vi "IO_TEST_TankControl18V7.vi"() -> ()   [LabVIEW 2024]
uses:
  Control Definitions/Def_Status18v7.ctl
  <vilib>/Instr/_visa.llb/VISA Configure Serial Port (Instr).vi
  LabVIEW_InstrDriver_forLK-G3000_ver1_0_1_0/32bit/Keyence LK-G3000/Keyence LK-G3000.lvlib
panel:
  out "Elapsed":dbl format="%#.2g"
  out "Rate In/sec":dbl=nan format="%#.4g"
  in  "Reset":bool
  in  "Start":bool
  in  "Time (sec)":dbl=30.0
  in  "Laser ON":bool=TRUE
  out "Level PV":dbl(slide)=7.1220598220825195 scale=0.0..10.0
  out "Laser Raw":sgl=2.4953
  in  "Inputs":T1={"Fill!Drain"=TRUE, "Speed"=2, "Send Msg"=FALSE, "Write Buf"="GO"} {"Speed" scale=0.0..100.0}
  out "Outputs":T3={"Status"=[TRUE, FALSE, FALSE, FALSE, FALSE, FALSE, FALSE, FALSE, FALSE, FALSE, FALSE, FALSE, FALSE, FALSE, FALSE, FALSE, FALSE, FALSE, FALSE, FALSE, FALSE, FALSE, FALSE, FALSE, FALSE, FALSE, FALSE, FALSE, FALSE, FALSE, FALSE, FALSE], "Match"=-1, "Rx Speed"=".+64", "Tx"=FALSE}
  in  "Sens Reply":bool
  out "TX Buf":string="D0\r"
  in  "Send Reply":string
  out "read buffer ASC":string="!1\r\n"
  in  "Exit":bool
  # "Use this Timer section\nto measure the Level dl/dt"
  # "Laser ON When Laser\nis on Line."
  # "Use if off line to generate\na test Reply to Write msg"
  # "Fill"
  # "Drain"
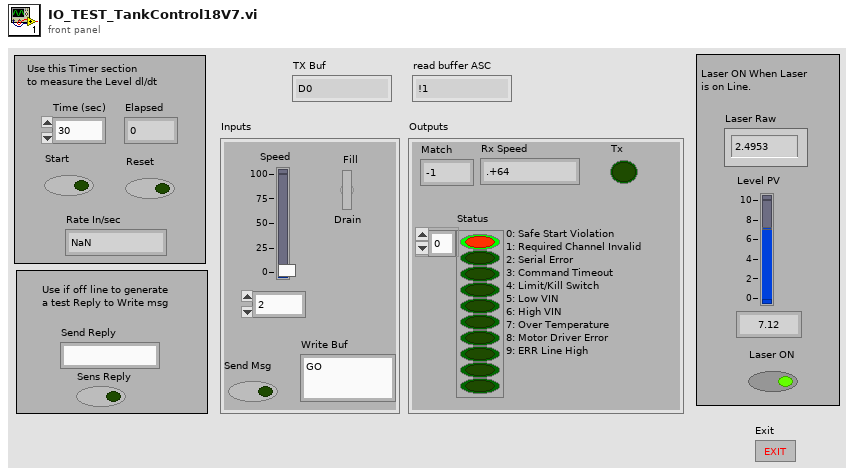
[diagram p1: front panel]
types:
  T1 = cluster{"Fill!Drain":bool, "Speed":i16, "Send Msg":bool, "Write Buf":string}
  T2 = typedef "Def_Status18v7.ctl" = bool[]
  T3 = cluster{"Status":T2, "Match":i32, "Rx Speed":string, "Tx":bool}
  T4 = typedef "Keyence LK-G3000.lvlib/LKIF_FLOATVALUE.ctl" = cluster{"LKIF_FLOATRESULT":T5, "Value":sgl}
  T5 = typedef "Keyence LK-G3000.lvlib/LKIF_FLOATRESULT.ctl" = i32
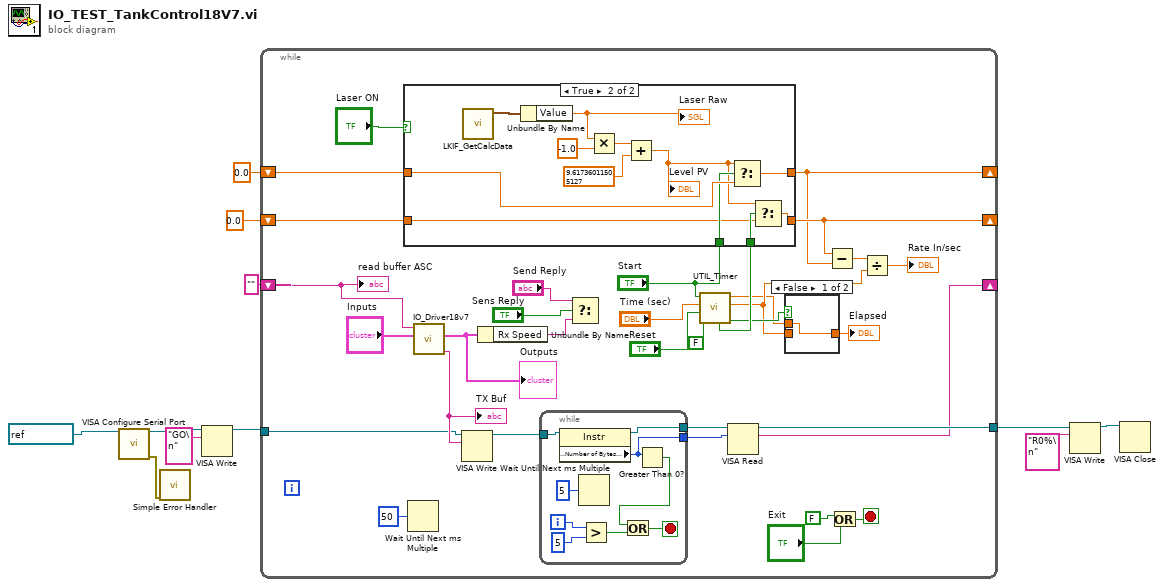
[diagram p0: block diagram]
diagram:
  n1 = call-poly "VISA Configure Serial Port"("VISA resource name"=refnum<visa-resource-name> "COM4") -> ("VISA resource name out"=w8:refnum<visa-resource-name>, "error out"=w9:errorcluster)  [unwired: 13 in]
  n2 = call <vilib>:"Simple Error Handler.vi"("error in (no error)"=w9) -> ()  [unwired: 4 in, 5 out]
  n3 = VISA Write(VISA resource name=w8, write buffer="GO\n") -> (VISA resource name out=w6:refnum<visa-resource-name>)  [unwired: 1 in, 2 out]
  n4 = while {
    shift-right: [w28] -> _
    shift-left: "" ("Repy") -> [w37]
    tunnel: w6 -> [w33]
    tunnel: [w29] -> w5
    shift-right: [w19] -> _
    shift-left: sgl 0.0 -> [w26]
    shift-right: [w20] -> _
    shift-left: sgl 0.0 -> [w22]
    stop <- w44 stop-if-true
    n5 = Wait Until Next ms Multiple(millisecond multiple=u32 50) -> ()  [unwired: 1 out]
    n6 = call "IO_Driver18v7.vi"("Inputs"="Inputs", "Reply In"=w37) -> ("Tx Buf Out"=w34:string, "Outputs"=w36:T3)  [unwired: 8 in]
    "TX Buf" <- w34
    "Outputs" <- w36
    n7 = VISA Write(VISA resource name=w33, write buffer=w34) -> (VISA resource name out=w32:refnum<visa-resource-name>)  [unwired: 1 in, 2 out]
    n8 = Unbundle By Name(w36) -> ("Rx Speed"=w35:string)
    n9 = while {
      tunnel: w32 -> [w68]
      tunnel: [w62] -> w31
      tunnel: [w61] -> w30
      i -> [w65]
      stop <- w67 stop-if-true
      n10 = property class="Instr"(reference=w68) -> (reference out=w62:refnum<visa-resource-name>, "Serial Settings:Number of Bytes at Serial Port"=w61:u32)  [unwired: 1 in, 1 out]
      n11 = Wait Until Next ms Multiple(millisecond multiple=u32 5) -> ()  [unwired: 1 out]
      n12 = Greater?(x=w65, y=5) -> (0:w66:bool)
      n13 = Greater Than 0?(x=w61) -> (x > 0?=w63:bool)
      n14 = Or(x=w63, y=w66) -> (x .or. y?=w67:bool)
    }
    n15 = Select(t="Send Reply", s="Sens Reply", f=w35) -> ()  [unwired: 1 out]
    n16 = call "UTIL_Timer.vi"("Auto Reset"=FALSE, "Reset"="Reset", "Time (sec)"="Time (sec)", "Start"="Start") -> ("Timed Out"=w15:bool, "Numeric 2"=w14:dbl, "Elapsed"=w12:dbl, "TO Trig"=w21:bool)  [unwired: 2 in, 2 out]
    n17 = case shown="True" "Laser ON" {
      tunnel: [w48 w55] -> w19
      tunnel: w26 -> [w48 w54]
      tunnel: "Start" -> [_ w53]
      tunnel: w21 -> [_ w52]
      tunnel: [w47 w51] -> w20
      tunnel: w22 -> [w47 w50]
      frame False {
      }
      frame True {
        n18 = call "LKIF_GetCalcData.vi"() -> ("CalcData1"=w60:T4)  [unwired: 9 in, 2 out]
        n19 = Unbundle By Name(w60) -> ("Value"=w59:sgl)
        "Laser Raw" <- w59
        n20 = Multiply(x=w59, y=sgl -1.0) -> (x*y=w57:sgl)
        n21 = Add(x=w57, y=sgl 9.61736) -> (x+y=w49:sgl)
        "Level PV" <- w49
        n22 = Select(t=w49, s=w53, f=w54) -> (s? t:f=w55:sgl)
        n23 = Select(t=w49, s=w52, f=w50) -> (s? t:f=w51:sgl)
      }
    }
    n24 = VISA Read(VISA resource name=w31, byte count=w30) -> (VISA resource name out=w29:refnum<visa-resource-name>, read buffer=w28:string)  [unwired: 1 in, 2 out]
    n25 = case shown="False" w15 {
      tunnel: w14 -> [_ w46]
      tunnel: [w45 w46] -> w13
      tunnel: w12 -> [w45 _]
      frame False {
      }
      frame True {
      }
    }
    "Elapsed" <- w13
    n26 = Subtract(x=w20, y=w19) -> (x-y=w18:sgl)
    n27 = Or(x=FALSE, y="Exit") -> (x .or. y?=w44:bool)
    n28 = Divide(x=w18, y=w14) -> (x/y=→"Rate In/sec":dbl)
    "read buffer ASC" <- w37
  }
  n29 = VISA Write(VISA resource name=w5, write buffer="R0%\n") -> (VISA resource name out=w4:refnum<visa-resource-name>)  [unwired: 1 in, 2 out]
  n30 = VISA Close(VISA resource name=w4) -> ()  [unwired: 1 in, 1 out]
